vi "Register PVs.vi"(8 "error in (no error)":errorcluster, 10 "Register Info":T1, 11 "CS++PVMonitor in":refnum<class "CS++PVMonitor.lvclass">) -> (0 "error out":errorcluster, 3 "CS++PVMonitor out":refnum<class "CS++PVMonitor.lvclass">)   [LabVIEW 2012, in "CS++PVMonitor.lvlib" / "CS++PVMonitor.lvclass"]
doc: "Register process variables."
uses:
  CS++PVMonitor.lvclass
  <vilib>/ActorFramework/Message Enqueuer/Message Enqueuer.lvclass
  CS++PVMonitor Messages/CS++PVUpdate Msg/CS++PVUpdate Msg.lvclass
  CS++PVMonitor.lvclass/CS++PVMonitor.ctl
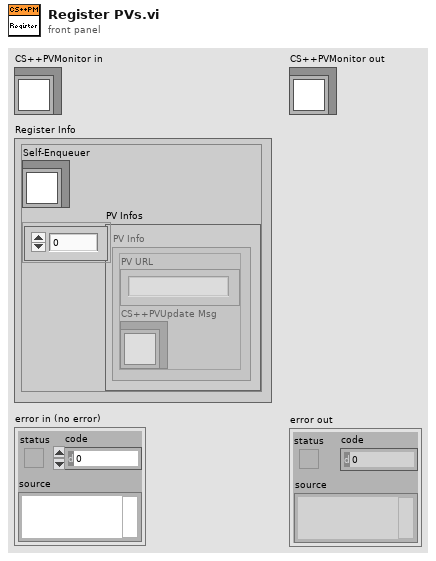
[diagram p1: front panel]
types:
  T1 = cluster{"Self-Enqueuer":refnum<class "Message Enqueuer.lvclass">, "PV Infos":cluster{"PV URL":string, "CS++PVUpdate Msg":refnum<class "CS++PVUpdate Msg.lvclass">}[]}
  T2 = cluster{"PV URL":string, "CS++PVUpdate Msg":refnum<class "CS++PVUpdate Msg.lvclass">}[]
  T3 = cluster{"PV URL":string, "Observers":cluster{"Enqueuer":refnum<class "Message Enqueuer.lvclass">, "CS++PVUpdate Msg":refnum<class "CS++PVUpdate Msg.lvclass">}[]}[]
  T4 = cluster{"PV URL":string, "Observers":cluster{"Enqueuer":refnum<class "Message Enqueuer.lvclass">, "CS++PVUpdate Msg":refnum<class "CS++PVUpdate Msg.lvclass">}[]}
  T5 = cluster{"Enqueuer":refnum<class "Message Enqueuer.lvclass">, "CS++PVUpdate Msg":refnum<class "CS++PVUpdate Msg.lvclass">}[]
  T6 = cluster{"Self-Enqueuer":refnum<class "Message Enqueuer.lvclass">, "CS++PVUpdate Msg":refnum<class "CS++PVUpdate Msg.lvclass">}
  T7 = cluster{"Self-Enqueuer":refnum<class "Message Enqueuer.lvclass">, "CS++PVUpdate Msg":refnum<class "CS++PVUpdate Msg.lvclass">}[]
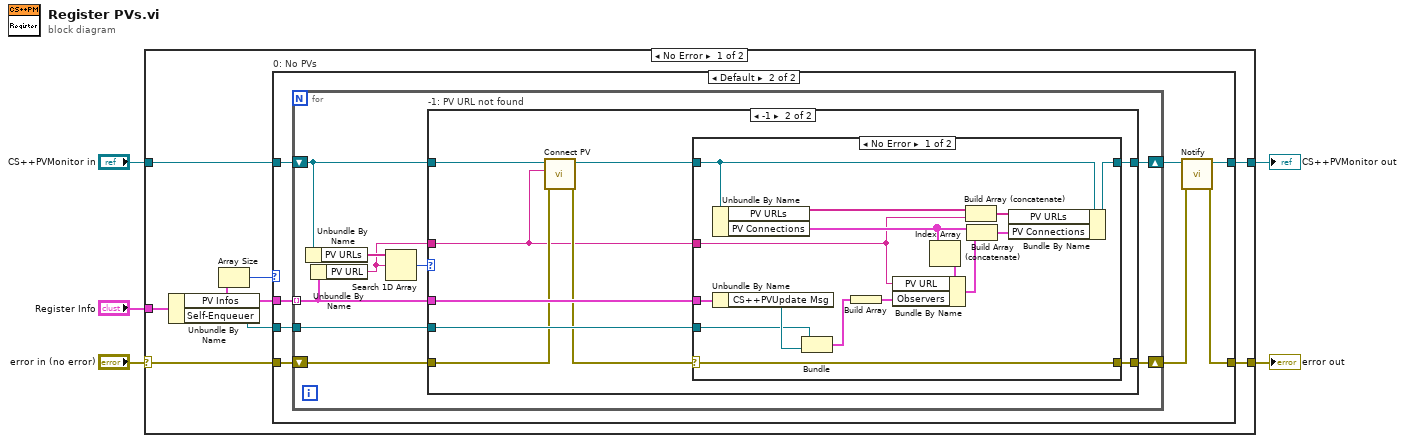
[diagram p0: block diagram]
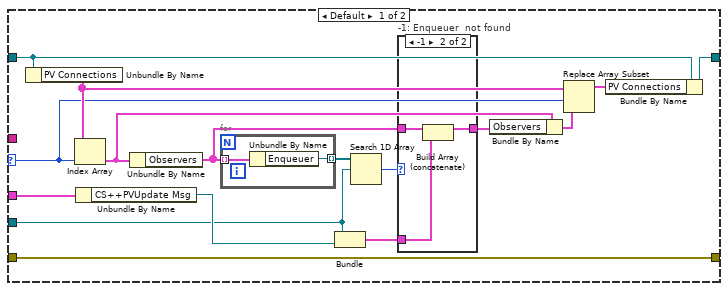
[diagram p3: hidden frame]
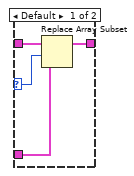
[diagram p4: hidden frame]
diagram:
  n1 = case shown="No Error" "error in (no error)" {
    selector: "error in (no error)" -> [w12 w85]
    tunnel: [w11 w85] -> w4
    tunnel: [w9 w84] -> w2
    tunnel: "CS++PVMonitor in" -> [w10 w84]
    tunnel: "Register Info" -> [w13 _]
    frame No Error {
      n2 = Unbundle By Name(w13) -> ("PV Infos"=w7:T2, "Self-Enqueuer"=w8:refnum<class "Message Enqueuer.lvclass">)
      n3 = Array Size(array=w7) -> (size(s)=w6:i32)
      n4 = case "0: No PVs" shown="Default" w6 {
        tunnel: w7 -> [_ w23]
        tunnel: w12 -> [w14 w22]
        tunnel: [w14 w16] -> w11
        tunnel: w10 -> [w15 w21]
        tunnel: [w15 w18] -> w9
        tunnel: w8 -> [_ w20]
        frame 0 {
        }
        frame Default {
          n5 = for {
            tunnel: w23 -> [w28] mode=indexing
            shift-right: [w26] -> w17
            shift-left: w22 -> [w25]
            shift-right: [w27] -> w19
            shift-left: w21 -> [w30]
            tunnel: w20 -> [w29]
            n6 = Unbundle By Name(w30) -> ("PV URLs"=w32:string[])
            n7 = Unbundle By Name(w28) -> ("PV URL"=w24:string)
            n8 = Search 1D Array(1D array=w32, element=w24) -> (index of element=w31:i32)  [unwired: 1 in]
            n9 = case "-1: PV URL not found" shown="-1" w31 {
              selector: w31 -> [w43 _]
              tunnel: w30 -> [w47 w62]
              tunnel: w29 -> [w39 w65]
              tunnel: w28 -> [w38 w64]
              tunnel: [w45 w66] -> w27
              tunnel: [w42 w63] -> w26
              tunnel: w25 -> [w42 w60]
              tunnel: w24 -> [_ w58]
              frame Default {
                n10 = Unbundle By Name(w47) -> ("PV Connections"=w44:T3)
                n11 = Index Array(array=w44, index=w43) -> (element=w41:T4)
                n12 = Unbundle By Name(w38) -> ("CS++PVUpdate Msg"=w40:refnum<class "CS++PVUpdate Msg.lvclass">)
                n13 = Unbundle By Name(w41) -> ("Observers"=w46:T5)
                n14 = for {
                  tunnel: w46 -> [w57] mode=indexing
                  tunnel: [w56] -> w48 mode=indexing
                  n15 = Unbundle By Name(w57) -> ("Enqueuer"=w56:refnum<class "Message Enqueuer.lvclass">)
                }
                n16 = Bundle("Self-Enqueuer"=w39, "CS++PVUpdate Msg"=w40) -> (w37:T6)  [unwired: 1 in]
                n17 = Search 1D Array(1D array=w48, element=w39) -> (index of element=w33:i32)  [unwired: 1 in]
                n18 = case "-1: Enqueuer  not found" shown="-1" w33 {
                  selector: w33 -> [w49 _]
                  tunnel: w46 -> [w52 w55]
                  tunnel: w37 -> [w51 w53]
                  tunnel: [w50 w54] -> w35
                  frame Default {
                    n19 = Replace Array Subset(array=w52, new element=w51, index=w49) -> (w50:T5)
                  }
                  frame -1 {
                    n20 = Build Array (concatenate)(w55, w53) -> (w54:T7)
                  }
                }
                n21 = Bundle By Name(cluster=w41, "Observers"=w35) -> (w34:T4)
                n22 = Replace Array Subset(array=w44, new element=w34, index=w43) -> (w36:T3)
                n23 = Bundle By Name(cluster=w47, "PV Connections"=w36) -> (w45:refnum<class "CS++PVMonitor.lvclass">)
              }
              frame -1 {
                n24 = call-dynamic "Connect PV.vi"("error in (no error)"=w60, "PV URL"=w58, "CS++PVMonitor in"=w62) -> ("error out"=w59:errorcluster, "CS++PVMonitor out"=w61:refnum<class "CS++PVMonitor.lvclass">)  [unwired: 7 in]
                n25 = case shown="No Error" w59 {
                  selector: w59 -> [w67 w82]
                  tunnel: [w81 w83] -> w66
                  tunnel: w65 -> [w77 _]
                  tunnel: w64 -> [w76 _]
                  tunnel: w61 -> [w71 w83]
                  tunnel: w58 -> [w69 _]
                  tunnel: [w67 w82] -> w63
                  frame No Error {
                    n26 = Unbundle By Name(w71) -> ("PV URLs"=w68:string[], "PV Connections"=w80:T3)
                    n27 = Unbundle By Name(w76) -> ("CS++PVUpdate Msg"=w78:refnum<class "CS++PVUpdate Msg.lvclass">)
                    n28 = Bundle("Self-Enqueuer"=w77, "CS++PVUpdate Msg"=w78) -> (w75:T6)  [unwired: 1 in]
                    n29 = Build Array(w75) -> (w73:T7)
                    n30 = Index Array(array=w80) -> (element=w79:T4)  [unwired: 1 in]
                    n31 = Bundle By Name(cluster=w79, "PV URL"=w69, "Observers"=w73) -> (w72:T4)
                    n32 = Build Array (concatenate)(w68, w69) -> (w70:string[])
                    n33 = Build Array (concatenate)(w80, w72) -> (w74:T3)
                    n34 = Bundle By Name(cluster=w71, "PV URLs"=w70, "PV Connections"=w74) -> (w81:refnum<class "CS++PVMonitor.lvclass">)
                  }
                  frame Error {
                  }
                }
              }
            }
          }
          n35 = call-dynamic "Notify.vi"("error in (no error)"=w17, "CS++PVMonitor in"=w19) -> ("error out"=w16:errorcluster, "CS++PVMonitor out"=w18:refnum<class "CS++PVMonitor.lvclass">)  [unwired: 8 in]
        }
      }
    }
    frame Error {
    }
  }
  "error out" <- w4
  "CS++PVMonitor out" <- w2
